vi "LabVIEW Dev Load Test.vi"() -> (0 "error out":errorcluster)   [LabVIEW 2011]
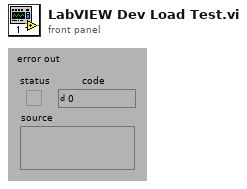
[diagram p1: front panel]
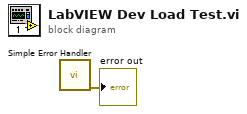
[diagram p0: block diagram]
diagram:
  n1 = call <vilib>:"Simple Error Handler.vi"() -> ("error out"=→"error out":errorcluster)  [unwired: 2 in, 7 out]
